vi "deser.ob.bools.vi"(11 "Numeric":u32 format="%.0b") -> (1 "Remove":bool, 2 "Edit":bool, 3 "Add":bool)   [LabVIEW 2020, in "fpganow.common.fpga.lvlib"]
uses:
  fpganow.common.fpga.lvlib
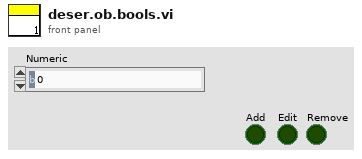
[diagram p1: front panel]
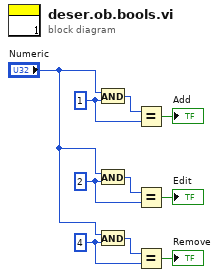
[diagram p0: block diagram]
diagram:
  w5 = u32 4 ("y")
  w7 = u32 2 ("y")
  w9 = u32 1 ("y")
  n1 = And(x="Numeric", y=w9) -> (x .and. y?=w10:u32)
  n2 = And(x="Numeric", y=w7) -> (x .and. y?=w8:u32)
  n3 = And(x="Numeric", y=w5) -> (x .and. y?=w6:u32)
  n4 = Equal?(x=w10, y=w9) -> (x = y?=→"Add":bool)
  n5 = Equal?(x=w8, y=w7) -> (x = y?=→"Edit":bool)
  n6 = Equal?(x=w6, y=w5) -> (x = y?=→"Remove":bool)
